vi "Mover4_Control_Inverse_Kinematics_Stream_Connection_No_Kinect.vi"() -> ()   [LabVIEW 2015]
uses:
  <vilib>/silver_ctls/ArrayMatrixCluster/Real Matrix NI_Silver.ctl
  <vilib>/Utility/miscctls.llb/LVRGBAColorTypeDef.ctl
  <vilib>/robotics/Kinematics/Analytical/6R/Type 1/Analytical Inverse Kinematics (6R Type 1).vi
  <vilib>/robotics/Kinematics/Robot/Forward Kinematics (Point).vi
  <vilib>/robotics/Kinematics/NI_Kinematics.lvlib
  <vilib>/robotics/Kinematics/Plotting/NI_Robotics_3DKinematics.lvlib
  <vilib>/robotics/Kinematics/Analytical/NI_Robotics_AnalyticKinematics.lvlib
  <vilib>/robotics/Kinematics/Analytical/6R/Type 1/NI_Robotics_6R Type 1 Serial Arm Class.lvclass
panel:
  out "Simulation":refnum<vi>(3d-picture)
  out "Motor positions (degree)":T1(array[cluster]) {"Error Code (bits)" format="%b"}
  in  "Choose solution":i32=6
  out "Joints positions to reach (degrees)":dbl[](array[numeric])
  out "End effector transform":T2 format="%#_3g"
  in  "Reset To Zero?":bool
  in  "x":dbl(slide) min=-0.4 max=0.4 step=0.01 scale=-0.4..0.4
  in  "y":dbl(slide) min=-0.4 max=0.4 step=0.01 scale=-0.4..0.4
  in  "z":dbl(slide) min=-0.4 max=0.6 step=0.01 scale=0.0..0.6 scale format="%#.2f"
  out "Position not reachable?":bool=TRUE
  in  "Target IP Address":string="172.22.11.2"
  in  "Stop":bool
  # "In the last column you can see the end \neffector coordinates (according to the theory). \nThis way, you can verify if the real robot reaches \nthis position correctly."
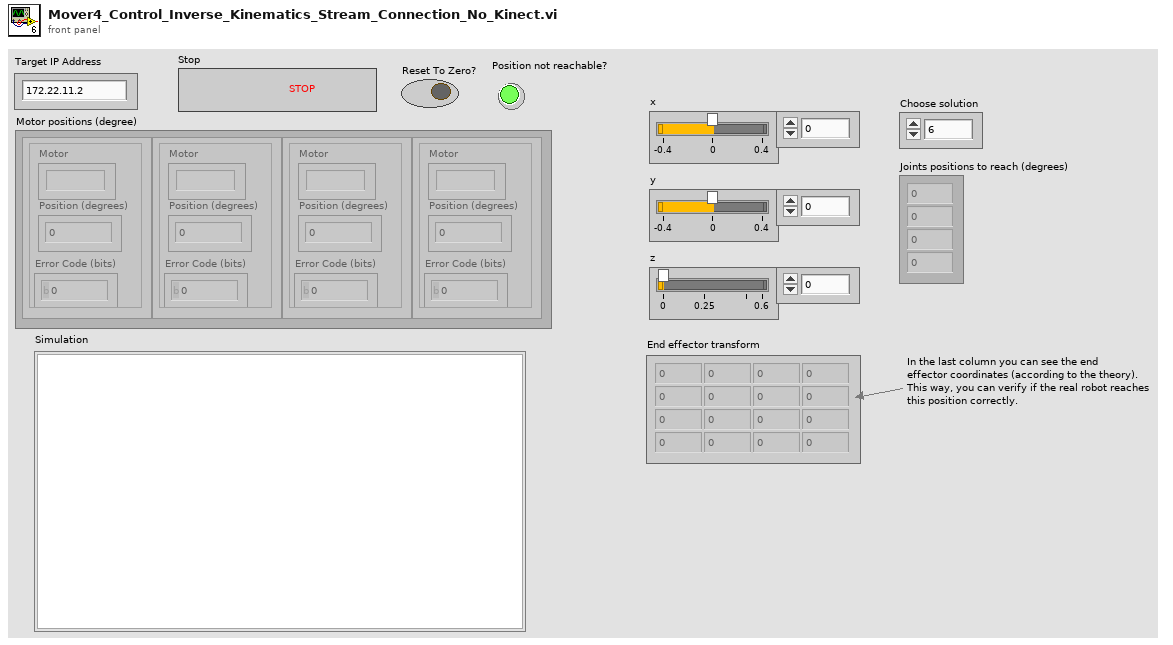
[diagram p1: front panel]
types:
  T1 = cluster{"Position (degrees)":i32, "Error Code (bits)":u8, "Motor":string}[]
  T2 = typedef "Real Matrix NI_Silver.ctl" = dbl[][]
  T3 = typedef "LVRGBAColorTypeDef.ctl" = cluster{"Red":sgl, "Green":sgl, "Blue":sgl, "Alpha":sgl}
  T4 = cluster{"Desired Position":u16, "Enable?":bool, "Reset?":bool}[]
  T5 = cluster{"ID":u8, "Position":u16, "Error Code":u8}[]
  T6 = cluster{"Read Access":enum8{"Allowed", "Required", "None"}, "Write Access":enum8{"Allowed", "Required", "None"}}
  T7 = typedef "NI_Matrix.lvlib/RealMatrix.ctl" = dbl[][]
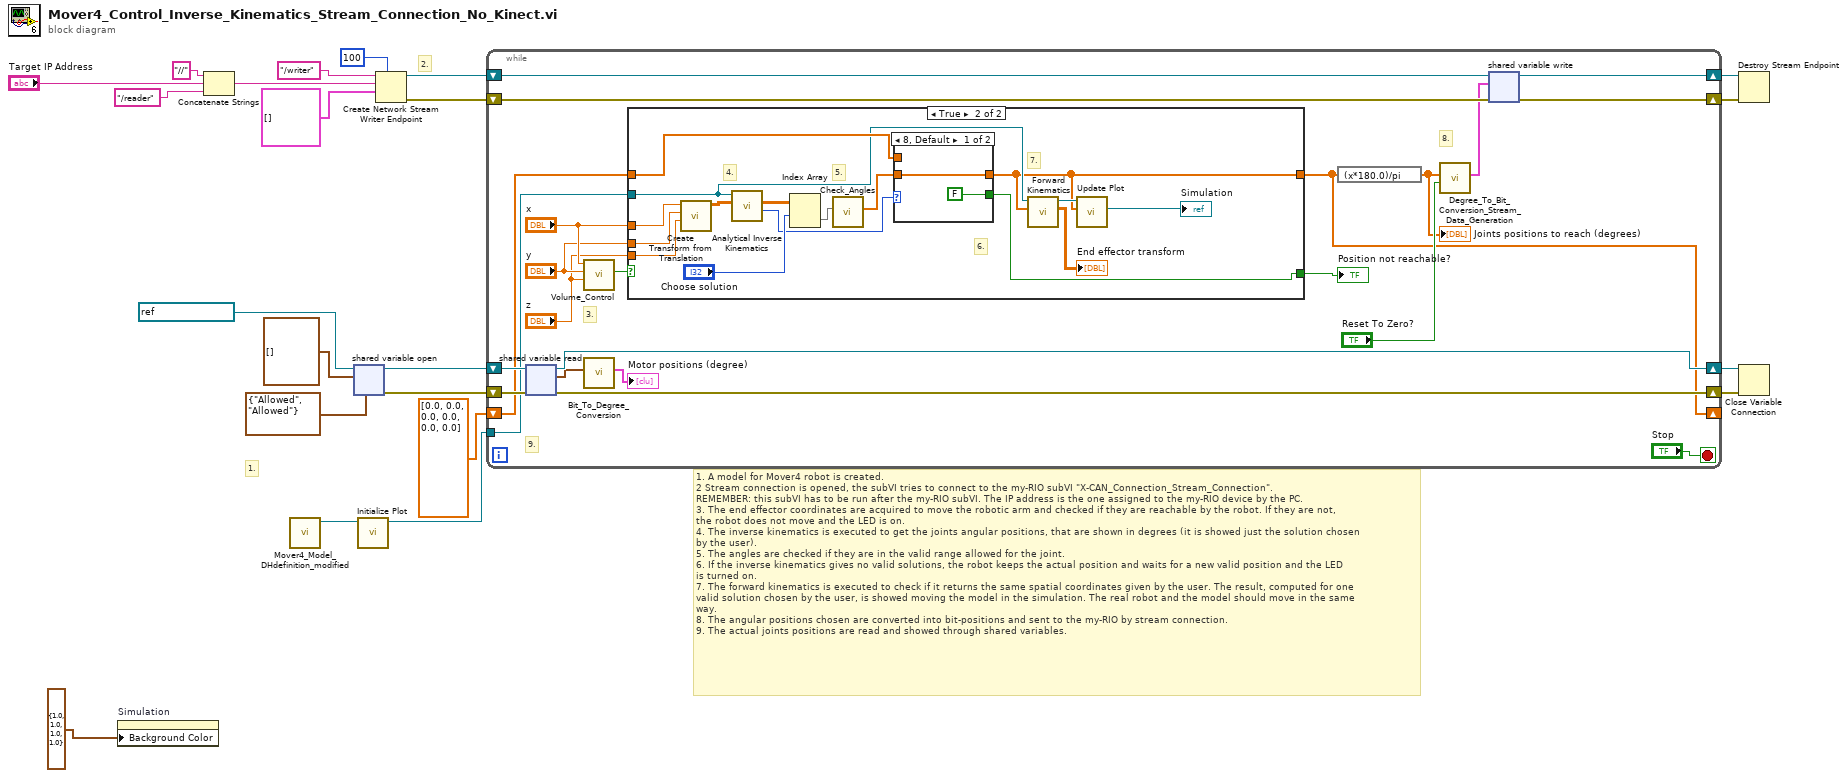
[diagram p0: block diagram]
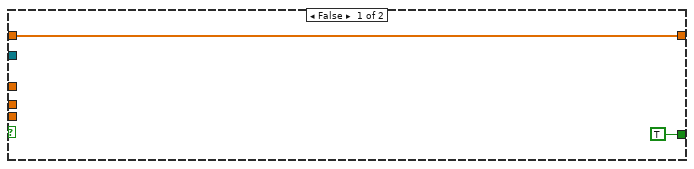
[diagram p2: hidden frame]
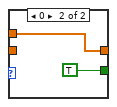
[diagram p3: hidden frame]
diagram:
  # "2."
  # "1."
  # "1. A model for Mover4 robot is created.\n2 Stream connection is opened, the subVI tries to connect to the my-RIO subVI \"X-CAN_Connection_Stream_Connection\".\nREMEMBER: this subVI has to be run after the my-RIO subVI. The IP address is the one assigned to the my-RIO device by the PC.\n3. The end effector coordinates are acquired to move the robotic arm and checked if they are reachable by the robot. If they are not,\nthe robot does not move and the LED is on.\n4. The inverse kinematics is executed to get the joints angular positions, that are shown in degrees (it is showed just the solution chosen\nby the user).\n5. The angles are checked if they are in the valid range allowed for the joint.\n6. If the inverse kinematics gives no valid solutions, the robot keeps the actual position and waits for a new valid position and the LED \nis turned on.\n7. The forward kinematics is executed to check if it returns the same spatial coordinates given by the user. The result, computed for one\nvalid solution chosen by the user, is showed moving the model in the simulation. The real robot and the model should move in the same \nway.\n8. The angular positions chosen are converted into bit-positions and sent to the my-RIO by stream connection.\n9. The actual joints positions are read and showed through shared variables."
  n1 = property on="Simulation" class="SceneGraphDisp (strict)"("Background Color"=T3 {"Red"=1.0, "Green"=1.0, "Blue"=1.0, "Alpha"=1.0}) -> ()  [unwired: 2 in, 2 out]
  n2 = Concatenate Strings("//", "Target IP Address", "/reader") -> (w15:string)
  n3 = call "Mover4_Model_DHdefinition_modified.vi"() -> ("serial arm out"=w2:refnum<class "NI_Robotics_6R Type 1 Serial Arm Class.lvclass">)  [unwired: 10 in, 1 out]
  n4 = shared-variable-open(refnum<k21> "ni.var.psp://stratom-myrio/Shared_Variables/New position" ("shared variable refnum in"), T5 [] ("New position 2"), T6 {"Read Access"=enum."Allowed", "Write Access"=enum."Allowed"} ("access")) -> (w22:refnum<k21>, w21:errorcluster)  [unwired: 1 in]
  n5 = call <vilib>:"Initialize Plot.vi"("serial arm in"=w2) -> ("serial arm out"=w3:refnum<class "NI_Robotics_6R Type 1 Serial Arm Class.lvclass">)  [unwired: 9 in, 1 out]
  n6 = Create Network Stream Writer Endpoint(7:100 ("writer buffer size"), 9:T4 [] ("Commands 2"), 10:w15, 11:"/writer" ("reader name")) -> (0:w8:errorcluster, 3:w9:refnum<k21>)  [unwired: 3 in]
  n7 = while {
    shift-right: [w42] -> w18
    shift-left: w22 -> [w44]
    shift-right: [w41] -> w17
    shift-left: w21 -> [w43]
    shift-right: [w37] -> w7
    shift-left: w9 -> [w39]
    shift-right: [w36] -> w6
    shift-left: w8 -> [w38]
    shift-right: [w27] -> _
    shift-left: dbl[] [0.0, 0.0, 0.0, 0.0, 0.0, 0.0] ("current joint positions") -> [w30]
    tunnel: w3 -> [w29]
    stop <- "Stop" stop-if-true
    # "9."
    # "8."
    # "3."
    n8 = shared-variable-read(w44, w43) -> (w42:refnum<k21>, w41:errorcluster, w24:T5)  [unwired: 1 out]
    n9 = call "Volume_Control.vi"("z (m)"="z", "y (m)"="y", "x (m)"="x") -> ("Range acceptable?"=w34:bool)  [unwired: 8 in]
    n10 = call "Bit_To_Degree_Conversion.vi"("Actual joints positions"=w24) -> ("Motor positions (degree)"=→"Motor positions (degree)":T1)  [unwired: 10 in]
    n11 = case shown="True" w34 {
      tunnel: "x" -> [_ w62]
      tunnel: "y" -> [_ w61]
      tunnel: "z" -> [_ w60]
      tunnel: [w46 w53] -> w27
      tunnel: [TRUE w59] -> w31
      tunnel: w30 -> [w46 w58]
      tunnel: w29 -> [_ w56]
      frame False {
      }
      frame True {
        # "7."
        # "6."
        # "5."
        # "4."
        n12 = call <vilib>:"Create Transform from Translation.vi"("z"=w60, "y"=w61, "x"=w62) -> ("transform"=w57:T7)  [unwired: 8 in]
        n13 = call-poly <vilib>:"Analytical Inverse Kinematics.vi"("end effector transform"=w57, "6R type 1 serial arm in"=w56) -> ("number of valid solutions"=w48:i32, "joint positions"=w52:T7)  [unwired: 6 in, 2 out]
        n14 = Index Array(array=w52, index (row)="Choose solution") -> (element=w50:dbl[])  [unwired: 1 in]
        n15 = call "Check_Angles.vi"("Joint positions (rad)"=w50) -> ("Adjusted joint positions (rad)"=w49:dbl[])  [unwired: 10 in]
        n16 = case shown="8, Default" w48 {
          tunnel: [w63 w65] -> w53
          tunnel: [FALSE TRUE] -> w59
          tunnel: w58 -> [_ w65]
          tunnel: w49 -> [w63 _]
          frame 8, Default {
          }
          frame 0 {
          }
        }
        n17 = call-poly <vilib>:"Forward Kinematics.vi"("joint positions"=w53, "serial arm in"=w56) -> ("end effector transform"=→"End effector transform":T7, "serial arm out"=w54:refnum<class "NI_Robotics_6R Type 1 Serial Arm Class.lvclass">)  [unwired: 7 in, 1 out]
        n18 = call <vilib>:"Update Plot.vi"("joint positions"=w53, "serial arm in"=w54) -> ("serial arm scene"=→"Simulation":refnum<vi>)  [unwired: 7 in, 2 out]
      }
    }
    "Position not reachable?" <- w31
    n19 = expression code="(x*180.0)/pi"(w27) -> (w26:dbl[])
    "Joints positions to reach (degrees)" <- w26
    n20 = call "Degree_To_Bit_Conversion_Stream_Data_Generation.vi"("Reset To Zero?"="Reset To Zero?", "Degree"=w26) -> ("Commands"=w35:T4)  [unwired: 9 in]
    n21 = shared-variable-write(w39, w38, w35) -> (w37:refnum<k21>, w36:errorcluster)  [unwired: 1 in, 1 out]
  }
  n22 = Destroy Stream Endpoint(8:w6, 11:w7) -> ()  [unwired: 1 out]
  n23 = Close Variable Connection(8:w17, 11:w18) -> ()  [unwired: 1 out]
